vi "Verify User.vi"(8 "error in (no error)":errorcluster, 9 "Account Data":T1, 10 "Verified?":bool, 11 "ATM Controller in":refnum<class "ATM Controller.lvclass">) -> (0 "error out":errorcluster, 3 "ATM Controller out":refnum<class "ATM Controller.lvclass">)   [LabVIEW 2020, in "ATM Controller.lvclass"]
uses:
  ATM Controller.lvclass
  Account Database/Account Data.ctl
  State.ctl
  ATM Controller.lvclass/ATM Controller.ctl
  Account Database/Account Database.lvclass
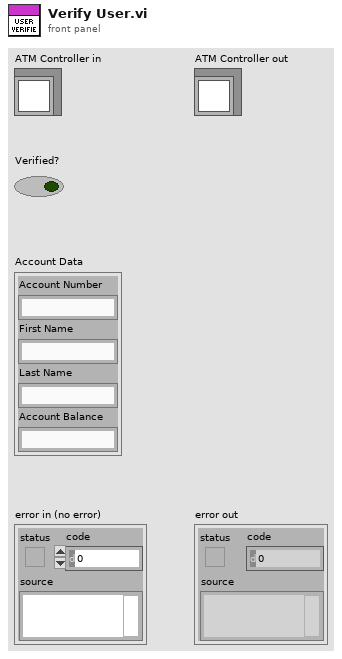
[diagram p1: front panel]
types:
  T1 = typedef "Account Database.lvclass/Account Data.ctl" = cluster{"Account Number":string, "First Name":string, "Last Name":string, "Account Balance":string}
  T2 = typedef "ATM Controller.lvclass/State.ctl" = enum16{"Start", "Card Inserted", "Verification Failed", "Verification Succeeded", "Depositing", "Depositing Completed", "Terminate"}
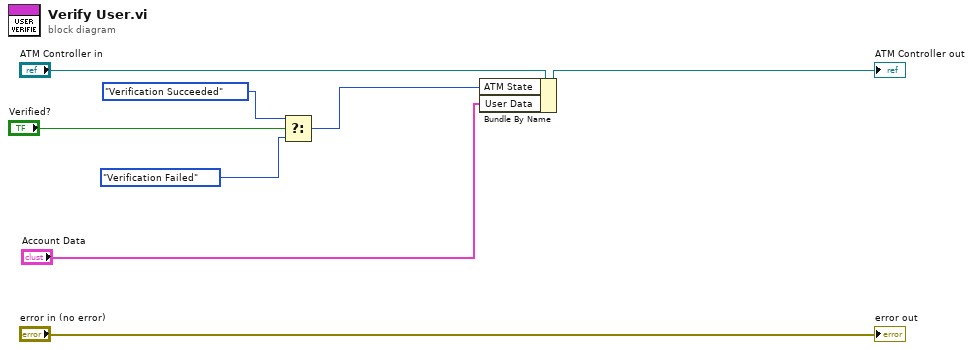
[diagram p0: block diagram]
diagram:
  n1 = Select(t=State."Verification Succeeded" ("ATM State"), s="Verified?", f=State."Verification Failed" ("ATM State")) -> (s? t:f=w2:T2)
  n2 = Bundle By Name(cluster="ATM Controller in", "ATM State"=w2, "User Data"="Account Data") -> (→"ATM Controller out":refnum<class "ATM Controller.lvclass">)
  "error out" <- "error in (no error)"
